vi "Chamber_Welcome Dialog.vi"() -> ()   [LabVIEW 2015]
doc: "TestStand Chamber example welcome dialog.\n____\nDelacor QMH Thermal Chamber Examples 4.0.0.21\nCopyright (c) 2018, Delacor"
panel:
  in  "Close":bool
  # "Welcome to the Delacor Queued Message Handler TestStand Thermal Chamber Controller Example.\n\nThis example executes using no process model file because there is no DUT.\n\nThe example contains one DQMH module - a Thermal Chamber Controller module that is written using the singleton form of the DQMH."
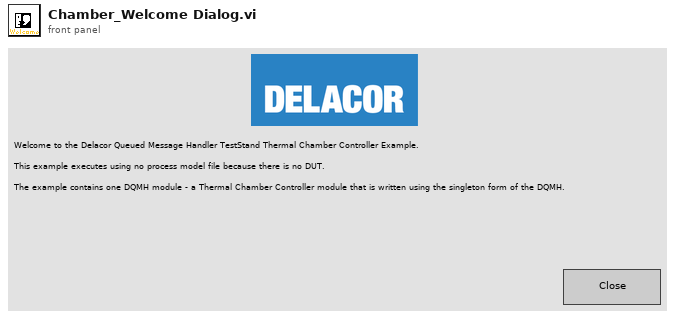
[diagram p1: front panel]
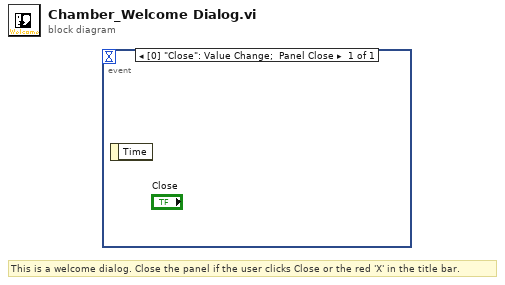
[diagram p0: block diagram]
diagram:
  # "This is a welcome dialog. Close the panel if the user clicks Close or the red 'X' in the title bar."
  n1 = event shown="[0] \"Close\": Value Change;  Panel Close" {
    selector: _ -> [_]
    dyn-events: _ -> [_]
    timeout: _ -> [_]
    event "Close": Value Change; Panel Close {
      n2 = event-data() -> ()  [unwired: 1 in, 1 out]
    }
  }
